vi "LVH5Iget_description.vi"(6 "error in (no error)":errorcluster, 9 "HDF5 Ref":T1) -> (0 "error out":errorcluster, 2 "Description":string, 3 "HDF5 Ref out":T1)   [LabVIEW 2017]
uses:
  <vilib>/UPVI/lvhdf5/library.llb/HDF5 Ref.ctl
panel:
  # "LVHDF5 Toolkit\nCopyright (c) 2005-2013 by Jason D. Sommerville\nCopyright (c) 2014 by UPVI, LLC.\n\nThis use and distribution of this file is governed by the terms found in \nLICENSE.txt distributed with this toolkit and installed at\n <user.lib>\\_lvhdf5\\LICENSE.txt"
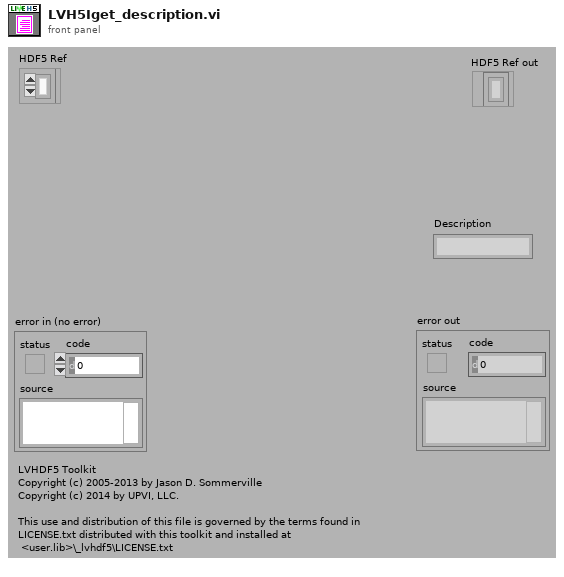
[diagram p1: front panel]
types:
  T1 = typedef "HDF5 Ref.ctl" = refnum<k1>
  T2 = enum32{"H5I_BADID", "H5I_FILE", "H5I_GROUP", "H5I_DATATYPE", "H5I_DATASPACE", "H5I_DATASET", "H5I_ATTR", "H5I_REFERENCE", "H5I_VFL", "H5I_GENPROP_CLS", "H5I_GENPROP_LST", "H5I_ERROR_CLASS", "H5I_ERROR_MSG", "H5I_ERROR_STACK"}
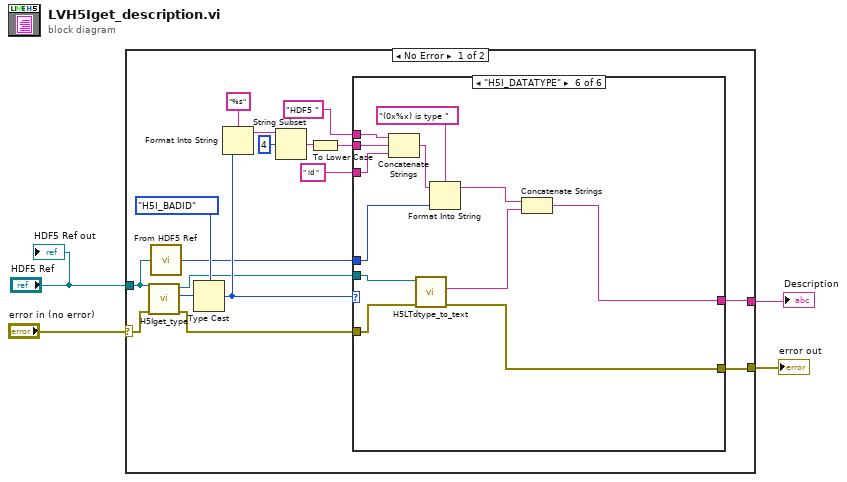
[diagram p0: block diagram]
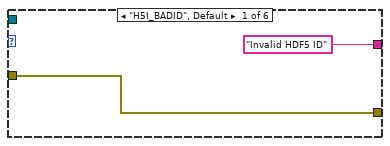
[diagram p2: hidden frame]
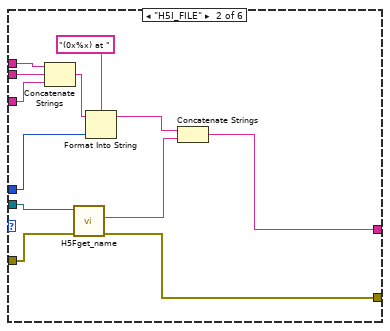
[diagram p3: hidden frame]
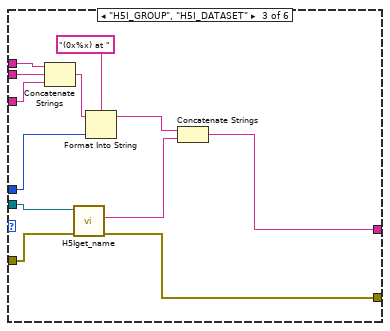
[diagram p4: hidden frame]
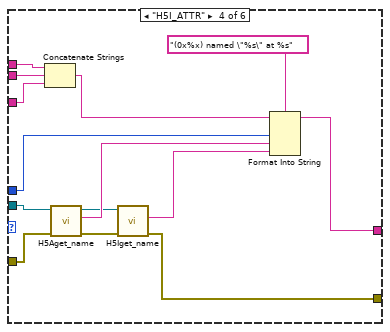
[diagram p5: hidden frame]
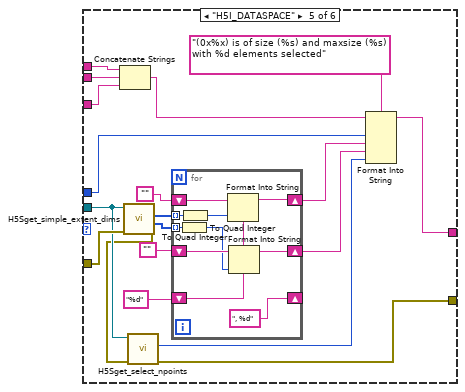
[diagram p6: hidden frame]
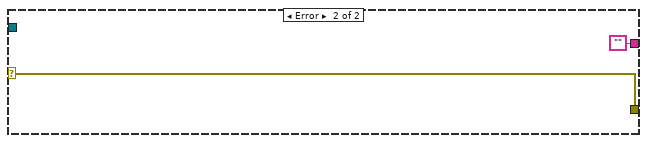
[diagram p7: hidden frame]
diagram:
  n1 = case shown="No Error" "error in (no error)" {
    selector: "error in (no error)" -> [w21 w104]
    tunnel: [w5 w104] -> w2
    tunnel: "HDF5 Ref" -> [w9 _]
    tunnel: [w12 ""] -> w1
    frame No Error {
      n2 = call <vilib>:"H5Iget_type.vi"("error in (no error)"=w21, "HDF5 Ref"=w9) -> ("error out"=w6:errorcluster, "Type"=w20:i32, "HDF5 Ref out"=w7:T1)  [unwired: 5 in]
      n3 = call <vilib>:"From HDF5 Ref.vi"("HDF5 Ref"=w9) -> ("I32"=w8:i32)
      n4 = Type Cast(type=T2."H5I_BADID" ("Type"), x=w20) -> (*(type *) &x=w17:T2)
      n5 = Format Into String(format string="%s", w17) -> (resulting string=w16:string)  [unwired: 2 in, 1 out]
      n6 = String Subset(string=w16, offset (0)=4) -> (substring=w14:string)  [unwired: 1 in]
      n7 = To Lower Case(string=w14) -> (all lower case string=w13:string)
      n8 = case shown="\"H5I_DATATYPE\"" w17 {
        tunnel: w13 -> [_ w35 w47 w61 w80 w102]
        tunnel: ["Invalid HDF5 ID" w25 w37 w54 w66 w95] -> w12
        tunnel: "HDF5 " ("format string") -> [_ w34 w46 w60 w79 w101]
        tunnel: " id " ("format string") -> [_ w33 w45 w59 w78 w100]
        tunnel: w8 -> [_ w32 w44 w58 w77 w99]
        tunnel: w7 -> [_ w29 w41 w52 w65 w94]
        tunnel: w6 -> [w22 w28 w40 w50 w74 w93]
        tunnel: [w22 w24 w36 w55 w63 w92] -> w5
        frame "H5I_BADID", Default {
        }
        frame "H5I_FILE" {
          n9 = Concatenate Strings(w34, w35, w33) -> (w31:string)
          n10 = call <vilib>:"H5Fget_name.vi"("error in (no error)"=w28, "HDF5 Attr Ref"=w29) -> ("error out"=w24:errorcluster, "Name"=w26:string)  [unwired: 5 in, 1 out]
          n11 = Format Into String(format string="(0x%x) at ", initial string=w31, w32) -> (resulting string=w27:string)  [unwired: 1 in, 1 out]
          n12 = Concatenate Strings(w27, w26) -> (w25:string)
        }
        frame "H5I_GROUP", "H5I_DATASET" {
          n13 = Concatenate Strings(w46, w47, w45) -> (w43:string)
          n14 = call <vilib>:"H5Iget_name.vi"("error in (no error)"=w40, "HDF5 Ref"=w41) -> ("error out"=w36:errorcluster, "Name"=w38:string)  [unwired: 4 in, 2 out]
          n15 = Format Into String(format string="(0x%x) at ", initial string=w43, w44) -> (resulting string=w39:string)  [unwired: 1 in, 1 out]
          n16 = Concatenate Strings(w39, w38) -> (w37:string)
        }
        frame "H5I_ATTR" {
          n17 = Concatenate Strings(w60, w61, w59) -> (w57:string)
          n18 = call <vilib>:"H5Aget_name.vi"("error in (no error)"=w50, "HDF5 Attr Ref"=w52) -> ("error out"=w49:errorcluster, "Name"=w51:string, "HDF5 Attr Ref out"=w48:T1)  [unwired: 5 in]
          n19 = call <vilib>:"H5Iget_name.vi"("error in (no error)"=w49, "HDF5 Ref"=w48) -> ("error out"=w55:errorcluster, "Name"=w53:string)  [unwired: 4 in, 2 out]
          n20 = Format Into String(format string="(0x%x) named \"%s\" at %s", initial string=w57, w58, w51, w53) -> (resulting string=w54:string)  [unwired: 1 in, 1 out]
        }
        frame "H5I_DATASPACE" {
          n21 = Concatenate Strings(w79, w80, w78) -> (w76:string)
          n22 = call <vilib>:"H5Sget_simple_extent_dims.vi"("error in (no error)"=w74, "HDF5 Space Ref"=w65) -> ("error out"=w64:errorcluster, "Max Dims"=w72:u64[], "Dims"=w73:u64[])  [unwired: 4 in, 1 out]
          n23 = call <vilib>:"H5Sget_select_npoints.vi"("error in (no error)"=w64, "HDF5 Space Ref"=w65) -> ("error out"=w63:errorcluster, "Count"=w62:i64)  [unwired: 5 in, 1 out]
          n24 = for {
            tunnel: w73 -> [w83] mode=indexing
            tunnel: w72 -> [w84] mode=indexing
            shift-right: [w89] -> w68
            shift-left: "" -> [w90]
            shift-right: [w87] -> w67
            shift-left: "" -> [w88]
            shift-right: [", %d" ("format string")] -> _
            shift-left: "%d" ("format string") -> [w85]
            n25 = To Quad Integer(1:w84) -> (0:w82:i64)
            n26 = To Quad Integer(1:w83) -> (0:w81:i64)
            n27 = Format Into String(format string=w85, initial string=w90, w81) -> (resulting string=w89:string)  [unwired: 1 in, 1 out]
            n28 = Format Into String(format string=w85, initial string=w88, w82) -> (resulting string=w87:string)  [unwired: 1 in, 1 out]
          }
          n29 = Format Into String(format string="(0x%x) is of size (%s) and maxsize (%s) with %d elements selected", initial string=w76, w77, w68, w67, w62) -> (resulting string=w66:string)  [unwired: 1 in, 1 out]
        }
        frame "H5I_DATATYPE" {
          n30 = Concatenate Strings(w101, w102, w100) -> (w98:string)
          n31 = call <vilib>:"H5LTdtype_to_text.vi"("error in (no error)"=w93, "HDF5 Type Ref"=w94) -> ("error out"=w92:errorcluster, "Text Description"=w91:string)  [unwired: 5 in, 1 out]
          n32 = Format Into String(format string="(0x%x) is type ", initial string=w98, w99) -> (resulting string=w96:string)  [unwired: 1 in, 1 out]
          n33 = Concatenate Strings(w96, w91) -> (w95:string)
        }
      }
    }
    frame Error {
    }
  }
  "error out" <- w2
  "Description" <- w1
  "HDF5 Ref out" <- "HDF5 Ref"
